vi "NameData_Get Array Data.vi"(8 "Error":errorcluster, 11 "Array Variant":variant) -> (0 "Error Out":errorcluster, 3 "Data Array Out":variant[](array[variant]), 5 "Names Out":string[](array[string]))   [LabVIEW 2020]
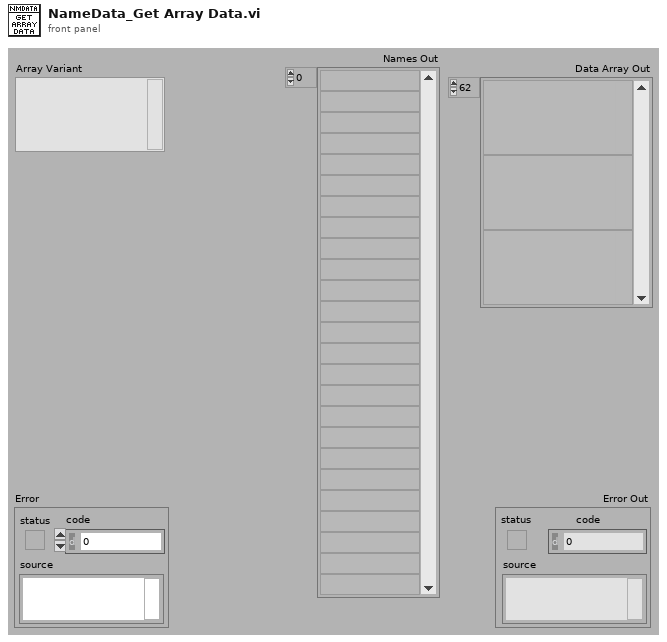
[diagram p1: front panel]
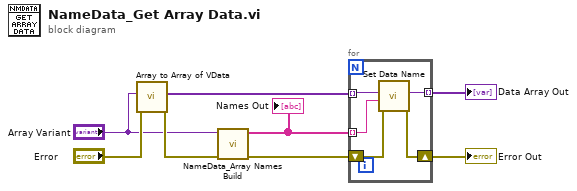
[diagram p0: block diagram]
diagram:
  n1 = call "Array to Array of VData.vi"("error in (no error)"="Error", "MultiD Array"="Array Variant") -> ("error out"=w7:errorcluster, "1D Array of Variants"=w5:variant[])  [unwired: 8 in]
  n2 = call "NameData_Array Names Build.vi"("Error"=w7, "Array Variant"="Array Variant") -> ("Error Out"=w2:errorcluster, "Name Array Out"=w4:string[])  [unwired: 8 in]
  "Names Out" <- w4
  n3 = for {
    tunnel: w5 -> [w13] mode=indexing
    tunnel: w4 -> [w12] mode=indexing
    tunnel: [w11] -> w3 mode=indexing
    shift-right: [w9] -> w1
    shift-left: w2 -> [w10]
    n4 = call "Set Data Name.vi"("error in (no error)"=w10, "Data Name"=w12, "Data"=w13) -> ("error out"=w9:errorcluster, "Renamed Data"=w11:variant)  [unwired: 7 in]
  }
  "Error Out" <- w1
  "Data Array Out" <- w3
